vi "compare_keys.vi"(10 "key (search)":T1, 11 "key (node)":T1) -> (2 "equal":bool, 3 "left_right":bool)   [LabVIEW 2015, in "binary_tree.lvlib"]
uses:
  binary_tree.lvlib
  _Controls/node_key.ctl
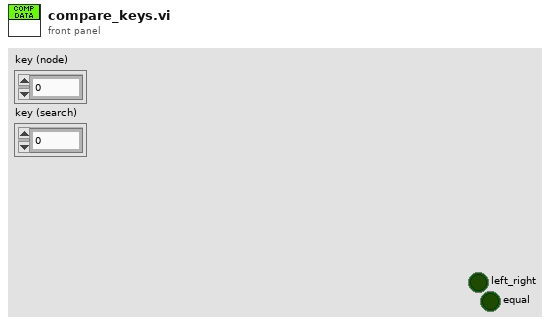
[diagram p1: front panel]
types:
  T1 = typedef "binary_tree.lvlib/node_key.ctl" = cluster{dbl}
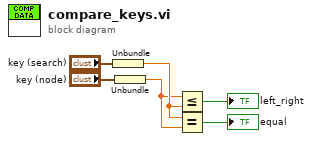
[diagram p0: block diagram]
diagram:
  n1 = Unbundle("key (search)") -> (w3:dbl)
  n2 = Unbundle("key (node)") -> (w2:dbl)
  n3 = Less Or Equal?(x=w2, y=w3) -> (x <= y?=→"left_right":bool)
  n4 = Equal?(x=w3, y=w2) -> (x = y?=→"equal":bool)
